vi "load class.vi"(8 "error in":errorcluster, 9 "available class paths":path[](array[path]), 10 "available class names":string[](array[string]), 11 "Class Name":string) -> (0 "error out":errorcluster, 3 "Object Out":refnum<class>)   [LabVIEW 2013, in "class discovery singleton.lvlib"]
doc: "Attempts to load a class, by name, either from memory or from disk. First it tries the exact name in memory. Then it tries the filename on disk. Then it tries an approximate match of all VIs in memory."
uses:
  class discovery singleton.lvlib
  NISE_CEF_TreeControl.lvlib
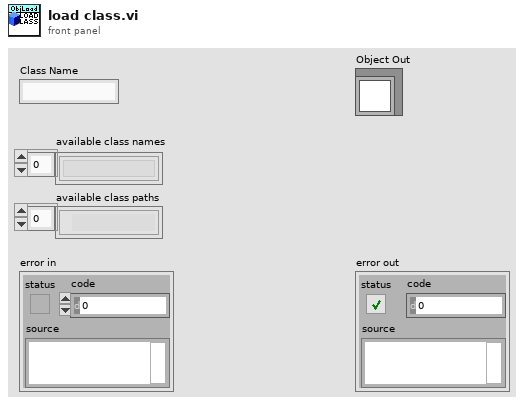
[diagram p1: front panel]
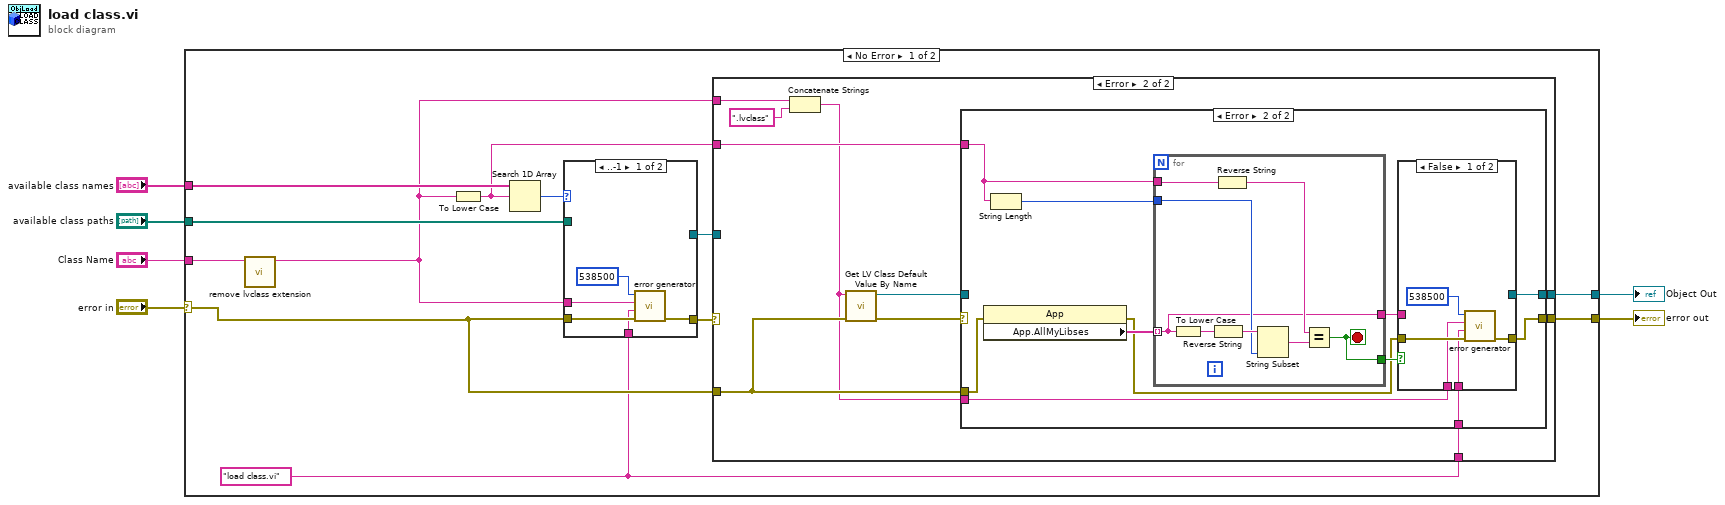
[diagram p0: block diagram]
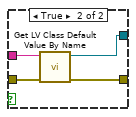
[diagram p4: hidden frame]
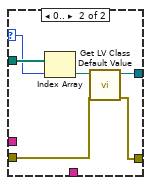
[diagram p5: hidden frame]
diagram:
  n1 = case shown="No Error" "error in" {
    selector: "error in" -> [w12 w72]
    tunnel: "Class Name" -> [w16 _]
    tunnel: [w15 _] -> w3
    tunnel: [w13 w72] -> w4
    tunnel: "available class paths" -> [w18 _]
    tunnel: "available class names" -> [w17 _]
    frame No Error {
      w7 = "load class.vi"
      n2 = call "remove lvclass extension.vi"("class name in"=w16) -> ("class name out"=w9:string)  [unwired: 10 in]
      n3 = To Lower Case(string=w9) -> (all lower case string=w8:string)
      n4 = Search 1D Array(1D array=w17, element=w8) -> (index of element=w11:i32)  [unwired: 1 in]
      n5 = case shown="..-1" w11 {
        selector: w11 -> [_ w67]
        tunnel: [w64 w71] -> w10
        tunnel: [_ w70] -> w14
        tunnel: w18 -> [_ w69]
        tunnel: w12 -> [w63 w66]
        tunnel: w9 -> [w62 _]
        tunnel: w7 -> [w61 _]
        frame ..-1 {
          n6 = call "error generator.vi"("error in"=w63, "source"=w61, "append error message"=w62, "error code (0)"=538500) -> ("error out"=w64:errorcluster)  [unwired: 5 in]
        }
        frame 0.. {
          n7 = Index Array(array=w69, index=w67) -> (element=w68:path)
          n8 = call <vilib>:"Get LV Class Default Value.vi"("error in (no error)"=w66, "class path"=w68) -> ("error out"=w71:errorcluster, "object"=w70:refnum<class>)  [unwired: 8 in]
        }
      }
      n9 = case shown="Error" w10 {
        selector: w10 -> [w19 _]
        tunnel: [w20 w30] -> w15
        tunnel: w14 -> [w20 _]
        tunnel: [w19 w29] -> w13
        tunnel: w9 -> [_ w27]
        tunnel: w12 -> [_ w28]
        tunnel: w8 -> [_ w23]
        tunnel: w7 -> [_ w21]
        frame No Error {
        }
        frame Error {
          n10 = Concatenate Strings(w27, ".lvclass" ("string")) -> (w22:string)
          n11 = call <vilib>:"Get LV Class Default Value By Name.vi"("error in (no error)"=w28, "class name"=w22) -> ("error out"=w25:errorcluster, "object"=w24:refnum<class>)  [unwired: 8 in]
          n12 = case shown="Error" w25 {
            selector: w25 -> [w32 _]
            tunnel: [w31 w36] -> w30
            tunnel: [w32 w37] -> w29
            tunnel: w28 -> [_ w43]
            tunnel: w22 -> [_ w35]
            tunnel: w24 -> [w31 _]
            tunnel: w23 -> [_ w34]
            tunnel: w21 -> [_ w33]
            frame No Error {
            }
            frame Error {
              n13 = property class="App"(error in=w43) -> (error out=w38:errorcluster, "App.AllMyLibses"=w42:string[])  [unwired: 1 in, 1 out]
              n14 = String Length(string=w34) -> (length=w41:i32)
              n15 = for {
                tunnel: w42 -> [w53] mode=indexing
                tunnel: w34 -> [w60]
                tunnel: w41 -> [w58]
                tunnel: [w53] -> w40
                tunnel: [w55] -> w39
                stop <- w55 stop-if-true
                n16 = To Lower Case(string=w53) -> (all lower case string=w54:string)
                n17 = Reverse String(1:w54) -> (0:w59:string)
                n18 = Reverse String(1:w60) -> (0:w56:string)
                n19 = String Subset(string=w59, length (rest)=w58) -> (substring=w57:string)  [unwired: 1 in]
                n20 = Equal?(x=w56, y=w57) -> (x = y?=w55:bool)
              }
              n21 = case shown="False" w39 {
                tunnel: w40 -> [_ w52]
                tunnel: w38 -> [w46 w51]
                tunnel: [w47 w50] -> w37
                tunnel: [_ w49] -> w36
                tunnel: w35 -> [w45 _]
                tunnel: w33 -> [w44 _]
                frame False {
                  n22 = call "error generator.vi"("error in"=w46, "source"=w44, "append error message"=w45, "error code (0)"=538500) -> ("error out"=w47:errorcluster)  [unwired: 5 in]
                }
                frame True {
                  n23 = call <vilib>:"Get LV Class Default Value By Name.vi"("error in (no error)"=w51, "class name"=w52) -> ("error out"=w50:errorcluster, "object"=w49:refnum<class>)  [unwired: 8 in]
                }
              }
            }
          }
        }
      }
    }
    frame Error {
    }
  }
  "error out" <- w4
  "Object Out" <- w3
